vi "sub_pf_observation.vi"(8 "rf_id":cluster{"x":dbl, "y":dbl}[](array[cluster]), 9 "u":T1, 10 "xd":T1, 11 "x_true":T1) -> (0 "ud":T1, 1 "xd out":T1, 2 "z":T1, 3 "x_true out":T1)   [LabVIEW 2019]
uses:
  <vilib>/Analysis/Matrix/Datatypes/RealMatrix.ctl
  Ctrl/cmd_common.ctl
  <vilib>/Analysis/Matrix/NI_Matrix.lvlib
  <vilib>/ptbypt/NI_PtbyPt.lvlib
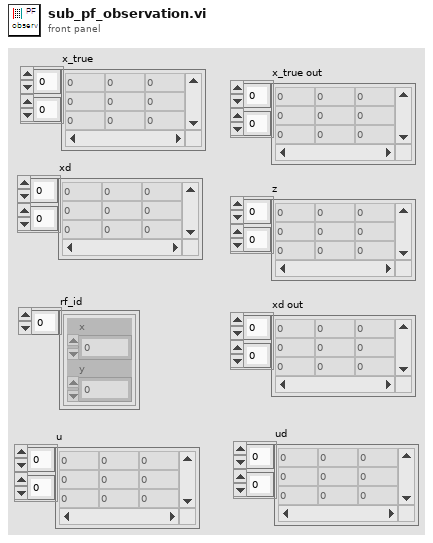
[diagram p1: front panel]
types:
  T1 = typedef "NI_Matrix.lvlib/RealMatrix.ctl" = dbl[][]
  T2 = typedef "cmd_common.ctl" = enum16{"read", "write"}
  T3 = cluster{"DT":dbl, "SIM_TIME":dbl, "MAX_RANGE":dbl, "NP":u32, "NTh":u32, "Q":T1, "R":T1, "Q_sim":T1, "R_sim":T1, "rf_id":cluster{"x":dbl, "y":dbl}[]}
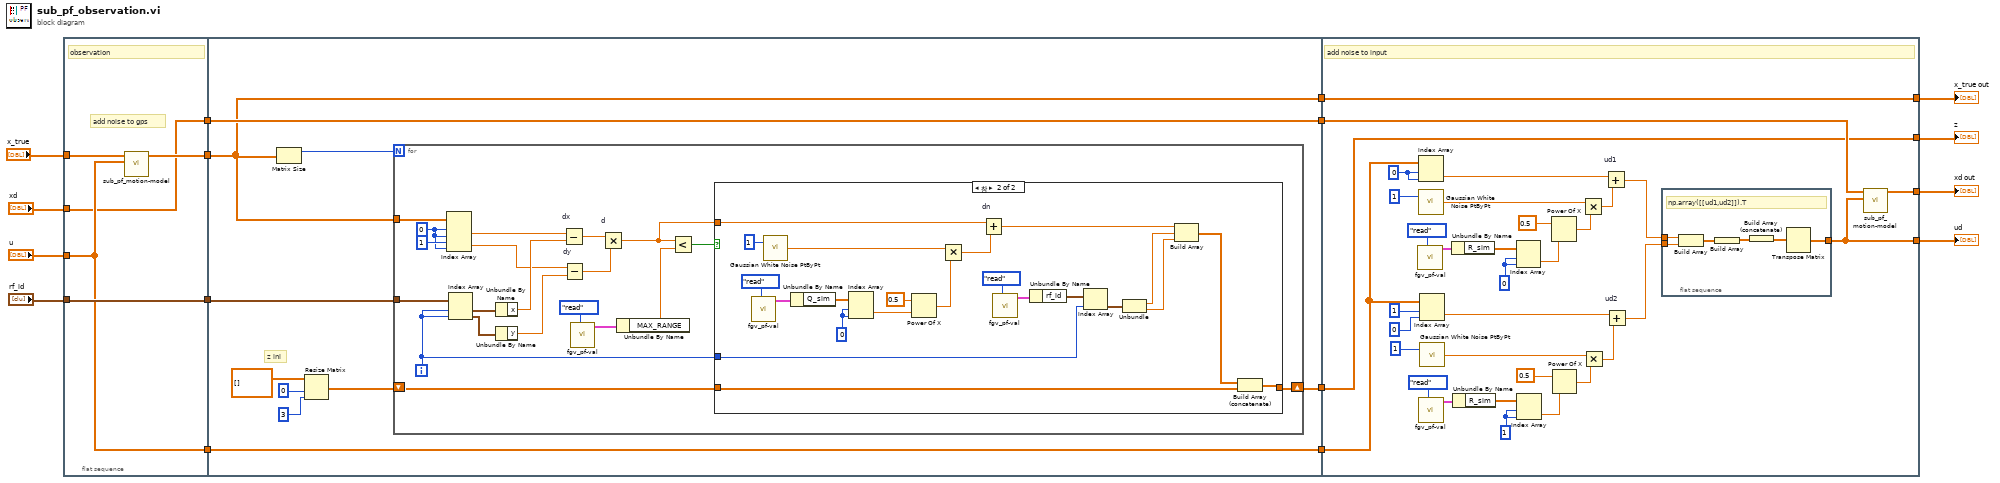
[diagram p0: block diagram]
diagram:
  n1 = flat-sequence {
    tunnel: "u" -> [w18]
    tunnel: [w21] -> w16
    tunnel: "x_true" -> [w19]
    tunnel: "rf_id" -> [w21]
    tunnel: [w17] -> w15
    tunnel: [w18] -> w14
    tunnel: [w20] -> w13
    tunnel: "xd" -> [w17]
    tunnel: w16 -> [w30]
    tunnel: [w23] -> w12
    tunnel: [w29] -> w11
    tunnel: w15 -> [w28]
    tunnel: [w28] -> w10
    tunnel: [w22] -> w9
    tunnel: w14 -> [w23]
    tunnel: w13 -> [w22]
    tunnel: w12 -> [w82]
    tunnel: [w79] -> w2
    tunnel: [w78] -> w3
    tunnel: w11 -> [w75]
    tunnel: [w75] -> w4
    tunnel: w10 -> [w77]
    tunnel: w9 -> [w76]
    tunnel: [w76] -> w6
    frame #0 {
      # "add noise to gps"
      # "observation"
      n2 = call "sub_pf_motion-model.vi"("u"=w18, "x_true"=w19) -> ("x_true out"=w20:T1)  [unwired: 9 in]
    }
    frame #1 {
      # "z ini"
      n3 = Matrix Size(0:w22) -> (1:w31:i32)  [unwired: 1 out]
      n4 = Resize Matrix(1:3 ("행의 개수"), 2:0 ("행의 개수"), 4:T1 [] ("행렬")) -> (0:w24:T1)
      n5 = for {
        N: w31 -> [_]
        tunnel: w30 -> [w49]
        shift-right: [w34] -> w29
        shift-left: w24 -> [w35]
        tunnel: w22 -> [w32]
        i -> [w33]
        w50 = 0 ("인덱스 (행)")
        n6 = Index Array(array=w32, index (row) #1=w50, index (col) #1=w50, index (row) #2=1 ("인덱스 (행)"), index (col) #2=w50) -> (element #1=w45:dbl, element #2=w44:dbl)
        n7 = Index Array(array=w49, index #1=w33, index #2=w33) -> (element #1=w48:cluster{"x":dbl, "y":dbl}, element #2=w47:cluster{"x":dbl, "y":dbl})
        n8 = Unbundle By Name(w48) -> ("x"=w46:dbl)
        n9 = Unbundle By Name(w47) -> ("y"=w43:dbl)
        n10 = Subtract "dx"(x=w45, y=w46) -> (x-y=w41:dbl)
        n11 = Subtract "dy"(x=w44, y=w43) -> (x-y=w42:dbl)
        n12 = call "fgv_pf-val.vi"("cmd"=cmd_common."read") -> ("pf-val out"=w39:T3)  [unwired: 10 in]
        n13 = Multiply "d"(x=w41, y=w42) -> (x*y=w36:dbl)
        n14 = Unbundle By Name(w39) -> ("MAX_RANGE"=w38:dbl)
        n15 = Less?(x=w36, y=w38) -> (x < y?=w37:bool)
        n16 = case shown="참" w37 {
          tunnel: w36 -> [_ w64]
          tunnel: w35 -> [w52 w54]
          tunnel: [w52 w53] -> w34
          tunnel: w33 -> [_ w59]
          frame False {
          }
          frame True {
            w70 = 0 ("인덱스 (행)")
            n17 = call "fgv_pf-val.vi"("cmd"=cmd_common."read") -> ("pf-val out"=w72:T3)  [unwired: 10 in]
            n18 = call <vilib>:"Gaussian White Noise PtByPt.vi"("standard deviation"=1 ("samples")) -> ("Gaussian white noise"=w66:dbl)  [unwired: 2 in]
            n19 = Unbundle By Name(w72) -> ("Q_sim"=w71:T1)
            n20 = Index Array(array=w71, index (row)=w70, index (col)=w70) -> (element=w69:dbl)
            n21 = Power Of X(1:w69, 2:0.5 ("y")) -> (0:w67:dbl)
            n22 = Multiply(x=w66, y=w67) -> (x*y=w65:dbl)
            n23 = Add "dn"(x=w64, y=w65) -> (x+y=w63:dbl)
            n24 = call "fgv_pf-val.vi"("cmd"=cmd_common."read") -> ("pf-val out"=w62:T3)  [unwired: 10 in]
            n25 = Unbundle By Name(w62) -> ("rf_id"=w60:cluster{"x":dbl, "y":dbl}[])
            n26 = Index Array(array=w60, index=w59) -> (element=w58:cluster{"x":dbl, "y":dbl})
            n27 = Unbundle(w58) -> ("x"=w57:dbl, "y"=w56:dbl)
            n28 = Build Array(w63, w57, w56) -> (w55:T1)
            n29 = Build Array (concatenate)(w55, w54) -> (w53:T1)
          }
        }
      }
    }
    frame #2 {
      w88 = 1 ("인덱스 (행)")
      w103 = 0 ("인덱스 (행)")
      w107 = 0 ("인덱스 (행)")
      # "add noise to input"
      n30 = call "fgv_pf-val.vi"("cmd"=cmd_common."read") -> ("pf-val out"=w104:T3)  [unwired: 10 in]
      n31 = Index Array(array=w82, index (row)=w107, index (col)=w107) -> (element=w96:dbl)
      n32 = call <vilib>:"Gaussian White Noise PtByPt.vi"("standard deviation"=1 ("samples")) -> ("Gaussian white noise"=w97:dbl)  [unwired: 2 in]
      n33 = call "fgv_pf-val.vi"("cmd"=cmd_common."read") -> ("pf-val out"=w87:T3)  [unwired: 10 in]
      n34 = Index Array(array=w82, index (row)=1 ("인덱스 (행)"), index (col)=0 ("인덱스 (행)")) -> (element=w95:dbl)
      n35 = call <vilib>:"Gaussian White Noise PtByPt.vi"("standard deviation"=1 ("samples")) -> ("Gaussian white noise"=w94:dbl)  [unwired: 2 in]
      n36 = Unbundle By Name(w104) -> ("R_sim"=w102:T1)
      n37 = Unbundle By Name(w87) -> ("R_sim"=w89:T1)
      n38 = Index Array(array=w102, index (row)=w103, index (col)=w103) -> (element=w99:dbl)
      n39 = Index Array(array=w89, index (row)=w88, index (col)=w88) -> (element=w92:dbl)
      n40 = Power Of X(1:w99, 2:0.5 ("y")) -> (0:w100:dbl)
      n41 = Power Of X(1:w92, 2:0.5 ("y")) -> (0:w91:dbl)
      n42 = Multiply(x=w97, y=w100) -> (x*y=w98:dbl)
      n43 = Multiply(x=w94, y=w91) -> (x*y=w93:dbl)
      n44 = Add "ud1"(x=w96, y=w98) -> (x+y=w81:dbl)
      n45 = Add "ud2"(x=w95, y=w93) -> (x+y=w80:dbl)
      n46 = flat-sequence {
        tunnel: w81 -> [w113]
        tunnel: w80 -> [w112]
        tunnel: [w108] -> w78
        frame #0 {
          # "np.array([[ud1,ud2]]).T"
          n47 = Build Array(w113, w112) -> (w111:dbl[])
          n48 = Build Array(w111) -> (w110:dbl[][])
          n49 = Build Array (concatenate)(w110) -> (w109:T1)
          n50 = Transpose Matrix(1:w109) -> (0:w108:T1)
        }
      }
      n51 = call "sub_pf_motion-model.vi"("u"=w78, "x_true"=w77) -> ("x_true out"=w79:T1)  [unwired: 9 in]
    }
  }
  "x_true out" <- w6
  "z" <- w4
  "ud" <- w3
  "xd out" <- w2
